vi "EventTouch_BallPossession.vi"(7 "Dist Para Toque":dbl=130.0, 8 "Tol para ang posse":dbl=0.3, 9 "Dist Para posse":dbl=180.0, 10 "IA State":T1={"our_robots"=[], "enemy_robots"=[], "balls"=[], "geometry"={"line_width"=0, "field_length"=0, "field_width"=0, "boundary_width"=0, "referee_width"=0, "goal_width"=0, "goal_depth"=0, "goal_wall_width"=0, "center_circle_radius"=0, "defense_radius"=0, "defense_stretch"=0, "free_kick_from_defense_dist"=0, "penalty_spot_from_field_line_dist"=0, "penalty_line_from_spot_dist"=0}, "IA Judge"={"stage"="", "command"="", "our_goalie_id"=0.0, "enemy_goalie_id"=0.0, "command enum"=enum."Halt", "Time"=enum."Azul"}, "Received Timestamp"=timestamp(0 s since 1904-01-01), "Events"={"Touch"=FALSE, "Ball out"=FALSE, "id touch"=0.0, "Ball out of \nVision"=FALSE, "Ball inside \nGoalie area"=FALSE, "Robot not responding"=FALSE, "Robots responding status"=[1.0, 1.0, 1.0, 1.0, 1.0, 1.0], "Enemy Ball \nPossession"=FALSE, "Pass State"=FALSE, "id end of pass"=0.0, "Kick"=FALSE, "Id Possession"=0.0}}) -> (0 "id touch":dbl, 1 "Toque":bool, 2 "id possesion":dbl, 3 "Posse inimigo":bool)   [LabVIEW 2016]
uses:
  Core/AI Input.ctl
  Core/AI Robot.ctl
  Intel/Functions Enum.ctl
  Intel/AttackerStates.ctl
  Core/AI Ball.ctl
  Core/Field Size.ctl
  Core/AI Judge.ctl
  Intel/Command Enum.ctl
  Events.ctl
  <vilib>/Analysis/coordinate.llb/Wrap Angle (scalar).vi
  <vilib>/Analysis/NI_AAL_Angle.lvlib
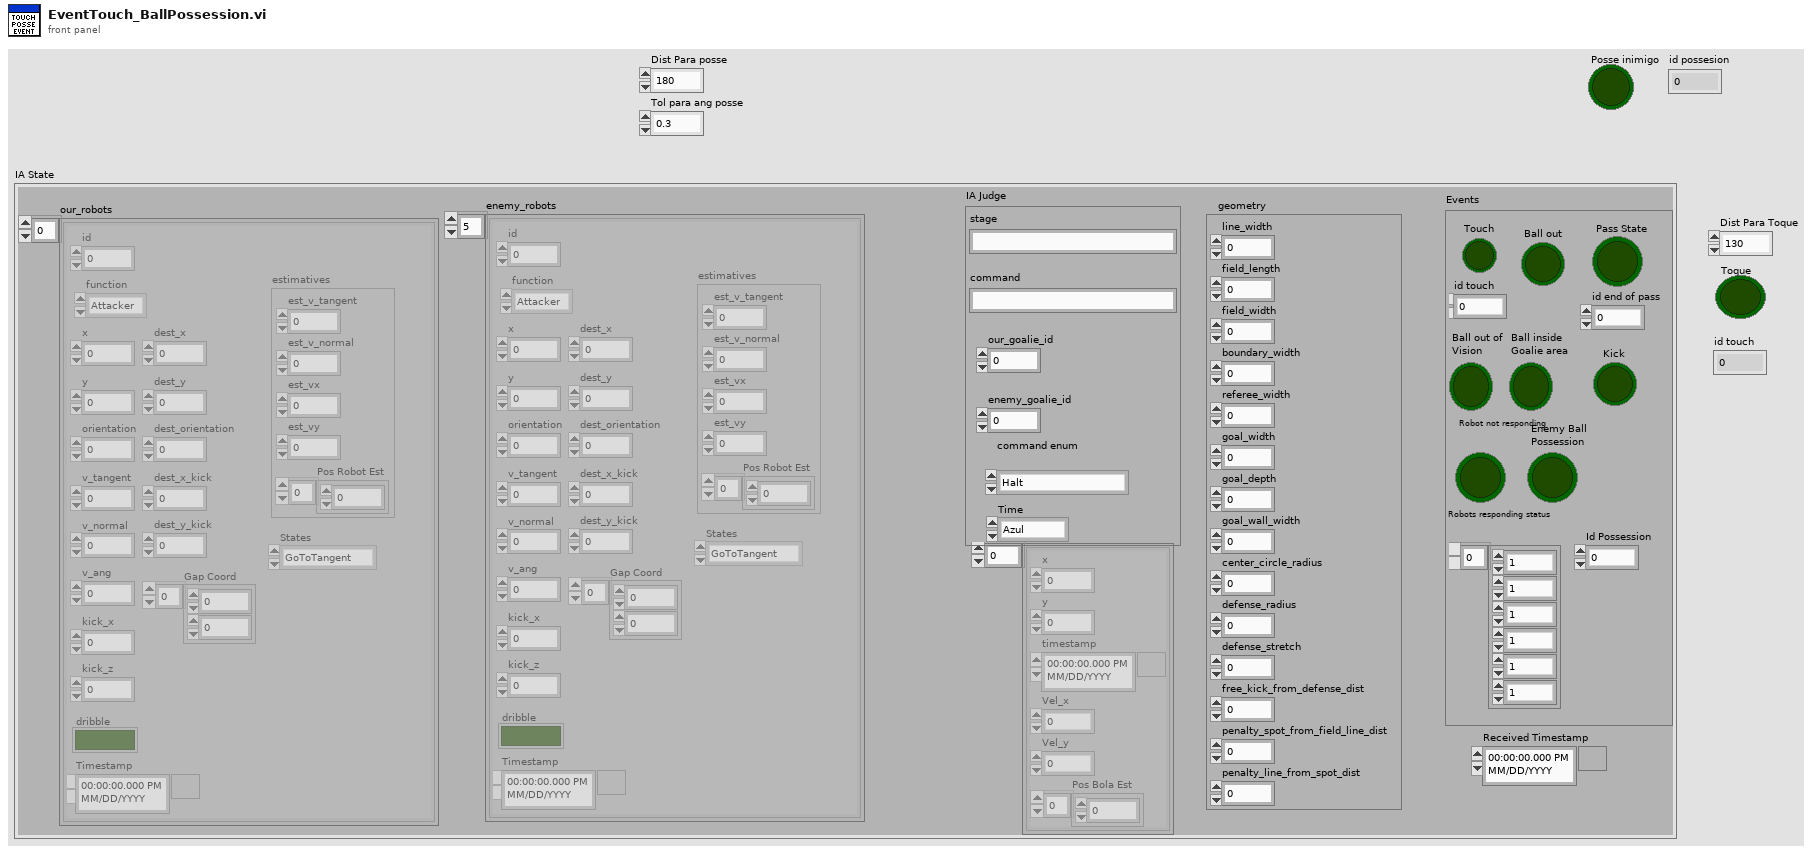
[diagram p1: front panel]
types:
  T1 = typedef "AI Input.ctl" = cluster{"our_robots":T2[], "enemy_robots":T2[], "balls":T5[], "geometry":T6, "IA Judge":T7, "Received Timestamp":timestamp, "Events":T9}
  T2 = typedef "AI Robot.ctl" = cluster{"id":u32, "function":T3, "x":dbl, "y":dbl, "orientation":dbl, "v_tangent":dbl, "v_normal":dbl, "v_ang":dbl, "kick_x":dbl, "kick_z":dbl, "dribble":bool, "Timestamp":timestamp, "dest_x":dbl, "dest_y":dbl, "dest_orientation":dbl, "estimatives":cluster{"est_v_tangent":dbl, "est_v_normal":dbl, "est_vx":dbl, "est_vy":dbl, "Pos Robot Est":dbl[]}, "dest_x_kick":dbl, "dest_y_kick":dbl, "Gap Coord":dbl[], "States":T4}
  T3 = typedef "Functions Enum.ctl" = enum16{"Attacker", "Goalie", "Defender", "Striker", "Goto 0", "Dummy", "Kicker", "ZigZag"}
  T4 = typedef "AttackerStates.ctl" = enum16{"Pass", "GoToTangent", "BallGetting", "GoToKick", ""}
  T5 = typedef "AI Ball.ctl" = cluster{"x":dbl, "y":dbl, "timestamp":timestamp, "Vel_x":dbl, "Vel_y":dbl, "Pos Bola Est":dbl[]}
  T6 = typedef "Field Size.ctl" = cluster{"line_width":u32, "field_length":u32, "field_width":u32, "boundary_width":u32, "referee_width":u32, "goal_width":u32, "goal_depth":u32, "goal_wall_width":u32, "center_circle_radius":u32, "defense_radius":u32, "defense_stretch":u32, "free_kick_from_defense_dist":u32, "penalty_spot_from_field_line_dist":u32, "penalty_line_from_spot_dist":u32}
  T7 = typedef "AI Judge.ctl" = cluster{"stage":string, "command":string, "our_goalie_id":dbl, "enemy_goalie_id":dbl, "command enum":T8, "Time":enum16{"Azul", "Amarelo"}}
  T8 = typedef "Command Enum.ctl" = enum16{"Halt", "Stop", "Force Start", "PKA Normal Start", "Prepare Kickoff Ally", "PKE Normal Start", "Prepare Kickoff Enemy", "Prepare Penalty Ally", "PPA Normal Start", "Prepare Penalty Enemy", "PPE Normal Start", "Direct Free Enemy", "Direct Free Ally", "Indirect Free Enemy", "Indirect Free Ally", "Timeout Enemy", "Timeout Ally", "Goal Enemy", "Goal Ally", "Ball Placement Enemy", "Ball Placement Ally", "Normal Half Time", "Extra Time Break", "Extra Half Time", "None"}
  T9 = typedef "Events.ctl" = cluster{"Touch":bool, "Ball out":bool, "id touch":dbl, "Ball out of \nVision":bool, "Ball inside \nGoalie area":bool, "Robot not responding":bool, "Robots responding status":dbl[], "Enemy Ball \nPossession":bool, "Pass State":bool, "id end of pass":dbl, "Kick":bool, "Id Possession":dbl}
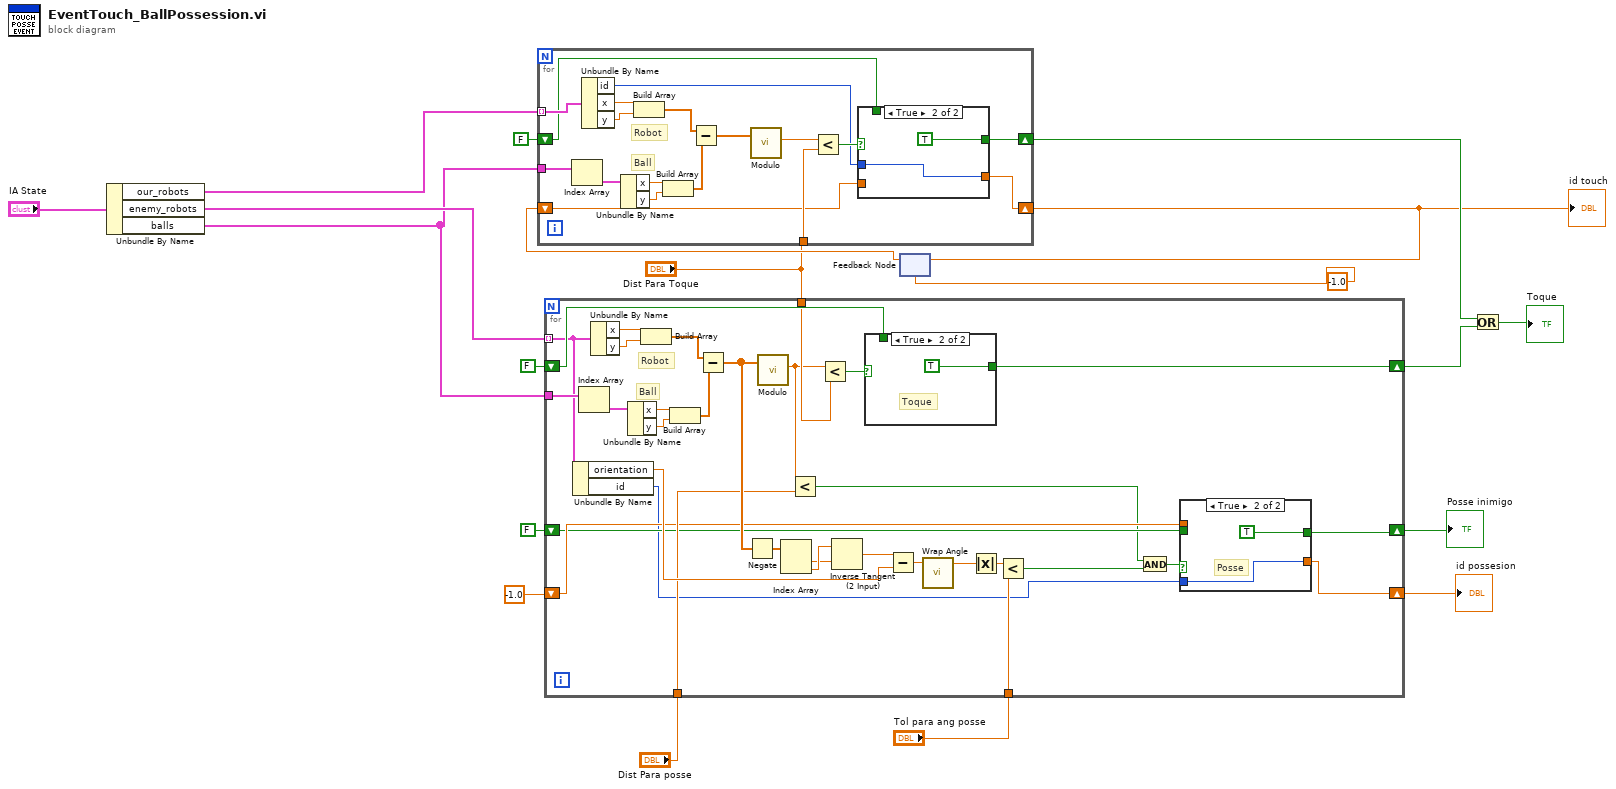
[diagram p0: block diagram]
diagram:
  n1 = Unbundle By Name("IA State") -> ("our_robots"=w11:T2[], "enemy_robots"=w15:T2[], "balls"=w14:T5[])
  n2 = for {
    tunnel: w15 -> [w41] mode=indexing
    tunnel: w14 -> [w52]
    shift-right: [w43] -> w13
    shift-left: FALSE -> [w42]
    tunnel: "Dist Para Toque" -> [w30]
    tunnel: "Tol para ang posse" -> [w33]
    shift-right: [w21] -> w1
    shift-left: -1.0 -> [w26]
    tunnel: "Dist Para posse" -> [w29]
    shift-right: [w25] -> w2
    shift-left: FALSE -> [w24]
    # "Ball"
    # "Robot"
    n3 = Unbundle By Name(w41) -> ("orientation"=w31:dbl, "id"=w20:u32)
    n4 = Index Array(array=w52) -> (element=w51:T5)  [unwired: 1 in]
    n5 = Unbundle By Name(w41) -> ("x"=w48:dbl, "y"=w47:dbl)
    n6 = Unbundle By Name(w51) -> ("x"=w50:dbl, "y"=w49:dbl)
    n7 = Build Array(w48, w47) -> (w46:dbl[])
    n8 = Build Array(w50, w49) -> (w45:dbl[])
    n9 = Subtract(x=w46, y=w45) -> (x-y=w32:dbl[])
    n10 = Negate(x=w32) -> (-x=w40:dbl[])
    n11 = call "Modulo.vi"("2D vector"=w32) -> ("Modulo"=w28:dbl)  [unwired: 10 in]
    n12 = Index Array(array=w40) -> (element #1=w38:dbl, element #2=w39:dbl)  [unwired: 2 in]
    n13 = Less?(x=w28, y=w29) -> (x < y?=w22:bool)
    n14 = Less?(x=w28, y=w30) -> (x < y?=w44:bool)
    n15 = Inverse Tangent (2 Input)(1:w38, 2:w39) -> (0:w37:dbl)
    n16 = case shown="True" w44 {
      tunnel: [w57 TRUE] -> w43
      tunnel: w42 -> [w57 _]
      frame False {
        # "Sem toque"
      }
      frame True {
        # "Toque"
      }
    }
    n17 = Subtract(x=w37, y=w31) -> (x-y=w36:dbl)
    n18 = call-poly <vilib>:"Wrap Angle.vi"("angle in"=w36) -> ("angle out"=w34:dbl)  [unwired: 9 in, 1 out]
    n19 = Absolute Value(x=w34) -> (abs(x)=w35:dbl)
    n20 = Less?(x=w35, y=w33) -> (x < y?=w23:bool)
    n21 = And(x=w22, y=w23) -> (x .and. y?=w27:bool)
    n22 = case shown="True" w27 {
      tunnel: [w53 TRUE] -> w25
      tunnel: w20 -> [_ w55]
      tunnel: [w54 w55] -> w21
      tunnel: w26 -> [w54 _]
      tunnel: w24 -> [w53 _]
      frame False {
        # "Sem toque"
      }
      frame True {
        # "Posse"
      }
    }
  }
  "Posse inimigo" <- w2
  "id possesion" <- w1
  n23 = feedback #1(-1.0) -> (w9:dbl)
  n24 = for {
    tunnel: w11 -> [w72] mode=indexing
    tunnel: w14 -> [w76]
    shift-right: [w64] -> w17
    shift-left: FALSE -> [w63]
    tunnel: "Dist Para Toque" -> [w62]
    shift-right: [w61] -> w10
    shift-left: w9 -> [w59]
    # "Ball"
    # "Robot"
    n25 = Index Array(array=w76) -> (element=w75:T5)  [unwired: 1 in]
    n26 = Unbundle By Name(w72) -> ("id"=w60:u32, "x"=w71:dbl, "y"=w70:dbl)
    n27 = Unbundle By Name(w75) -> ("x"=w74:dbl, "y"=w73:dbl)
    n28 = Build Array(w71, w70) -> (w69:dbl[])
    n29 = Build Array(w74, w73) -> (w68:dbl[])
    n30 = Subtract(x=w69, y=w68) -> (x-y=w67:dbl[])
    n31 = call "Modulo.vi"("2D vector"=w67) -> ("Modulo"=w65:dbl)  [unwired: 10 in]
    n32 = Less?(x=w65, y=w62) -> (x < y?=w66:bool)
    n33 = case shown="True" w66 {
      tunnel: [w78 TRUE] -> w64
      tunnel: w63 -> [w78 _]
      tunnel: [w77 w79] -> w61
      tunnel: w60 -> [_ w79]
      tunnel: w59 -> [w77 _]
      frame False {
      }
      frame True {
      }
    }
  }
  "id touch" <- w10
  n34 = feedback-in #1(w10) -> ()
  n35 = Or(x=w17, y=w13) -> (x .or. y?=→"Toque":bool)
